vi "ALP3 P.vi"(0 "Header Comments":string="This is a C(T) experiment being done in Physics 350.\r\nIt records the decay response of an RC circuit where the capacitance is a strong function of temperature.", 5 "Temperature Control Parameters":T2={"Start Temp"=30.0, "Temp Step"=10.0, "End Temp"=80.0} {"End Temp" format="%.2f"; "Temp Step" format="%.2f"; "Start Temp" format="%.2f"}, 9 "Timing Control Parameters":T1={"N cycles for averaging"=10, "N points per measurment"=1000, "Measurment time interval"=2e-05} {"Measurment time interval" format="%.2e"}, 11 "error in":errorcluster) -> (3 "Proceed":bool, 4 "data file path out":path, 6 "Temp Array":dbl[](array[numeric]), 10 "Timing Control Parameters out":T1={"N cycles for averaging"=10, "N points per measurment"=1000, "Measurment time interval"=2e-05} {"Measurment time interval" format="%.2e"}, 14 "Auto Launch Data Viewer at End":bool=TRUE, 15 "error out":errorcluster)   [LabVIEW 2016]
doc: "This vi runs when opened, aslo it can open a file, serach for specific numbers on the file to display them in the interface. Also, creates an array with the initail and final temp, and the temp step specified by the user. It can create a file with the data, it found in the file, includes the time, and it can include extra things that the user may want to include in the file. Also has the auto viewer and the data updates dynamically.\n\nAlexis Lopez\nP350\nCSUSB Physics"
uses:
  typedefs/temp control params.ctl
  typedefs/time control params.ctl
panel:
  in  "reload parameters":bool
  in  "exit":bool
  in  "create file and proceed":bool
  out "File Header":string="This is a C(T) experiment being done in Physics 350.\r\nIt records the decay response of an RC circuit where the capacitance is a strong function of temperature.\n\n2/14/2007\n1:53 PM\r\n\r\nStart temp = 30.0\r\nTemp step = 10.0\r\nEnd temp = 80.0\r\nNum temps = 6\r\nNum avg cycles = 10\r\nNum points per meas = 1000\r\nMeas time interval = 2.00E-5\n\nDDD\n\n"
  out "N temps":i32=6
  in  "Auto Launch Data Viewer at End":bool=TRUE
  # "Alexis Lopez\nP350\nCSUSB Physics"
  # "P350 C(T) Experimental Initialization"
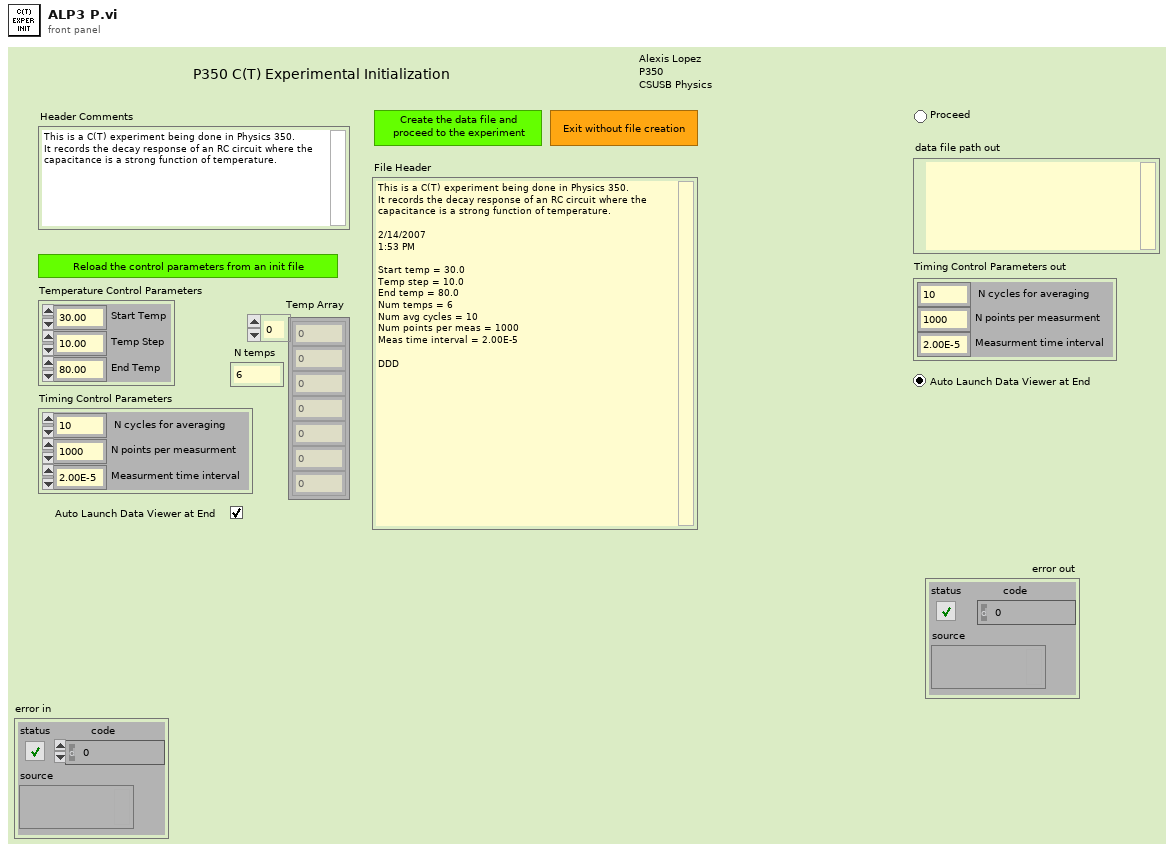
[diagram p1: front panel]
types:
  T1 = typedef "time control params.ctl" = cluster{"N cycles for averaging":i32, "N points per measurment":i32, "Measurment time interval":dbl}
  T2 = typedef "temp control params.ctl" = cluster{"Start Temp":dbl, "Temp Step":dbl, "End Temp":dbl}
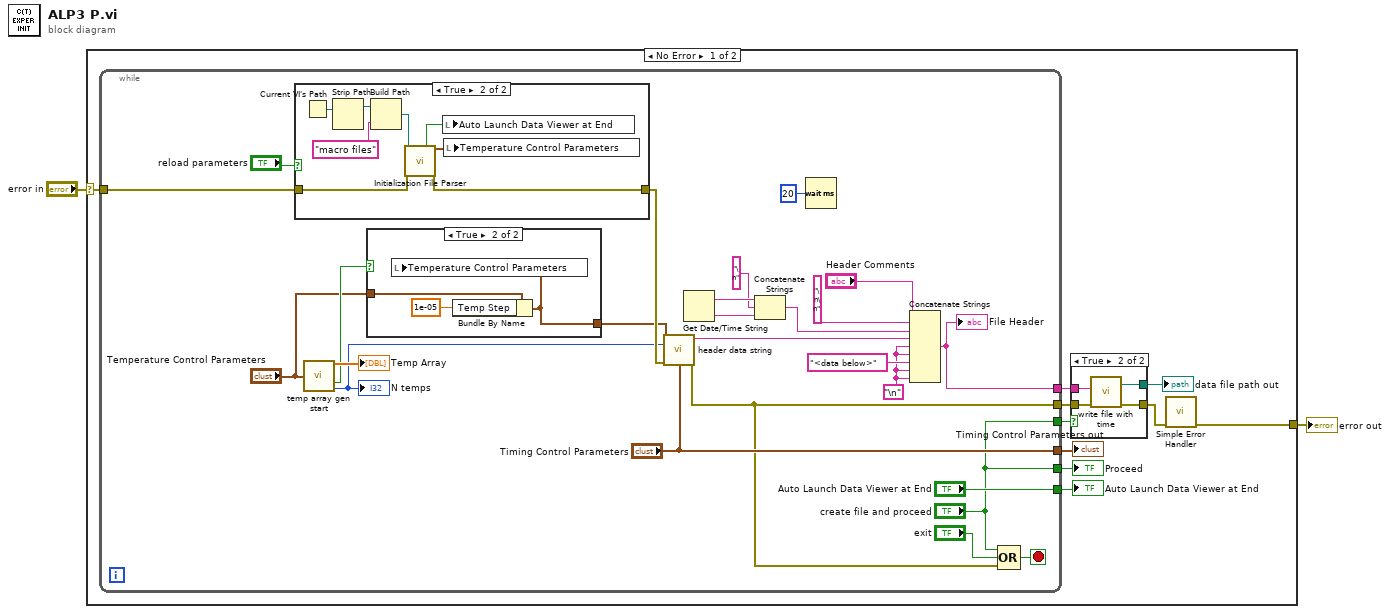
[diagram p0: block diagram]
diagram:
  n1 = case shown="No Error" "error in" {
    selector: "error in" -> [w12 w56]
    tunnel: [w3 w56] -> w1
    frame No Error {
      n2 = while {
        tunnel: [w42] -> w7
        tunnel: ["Auto Launch Data Viewer at End"] -> w10
        tunnel: ["Timing Control Parameters"] -> w11
        tunnel: ["create file and proceed"] -> w4
        tunnel: w12 -> [w34]
        tunnel: ["create file and proceed"] -> w9
        tunnel: [w29] -> w8
        stop <- w31 stop-if-true
        w37 = "\n"
        n3 = case shown="True" "reload parameters" {
          tunnel: w34 -> [w47 w55]
          tunnel: [w47 w54] -> w30
          frame False {
          }
          frame True {
            n4 = Current VI's Path() -> (path=w50:path)
            n5 = Strip Path(path=w50) -> (stripped path=w51:path)  [unwired: 1 out]
            n6 = Build Path(base path=w51, name or relative path="macro files") -> (appended path=w48:path)
            n7 = call "Initialization File Parser.vi"("path in"=w48, "error in"=w55) -> ("Auto Launch Data Viewer at End"=w52:bool, "temp control parameters"=w53:T2, "error out"=w54:errorcluster)  [unwired: 9 in, 2 out]
            n8 = local write "Auto Launch Data Viewer at End"(w52) -> ()
            n9 = local write "Temperature Control Parameters"(w53) -> ()
          }
        }
        n10 = call "temp array gen start.vi"("Temperature Control Parameters"="Temperature Control Parameters") -> ("Temp Array"=→"Temp Array":dbl[], "Warning time step too small"=w27:bool, "N temps"=w28:i32)  [unwired: 12 in]
        "N temps" <- w28
        n11 = case shown="True" w27 {
          tunnel: "Temperature Control Parameters" -> [w43 w46]
          tunnel: [w43 w44] -> w25
          frame False {
          }
          frame True {
            n12 = Bundle By Name(cluster=w46, "Temp Step"=1e-05) -> (w44:T2)
            n13 = local write "Temperature Control Parameters"(w44) -> ()
          }
        }
        n14 = call "header data string.vi"("Temperature Control Parameters"=w25, "N temps"=w28, "error in (no error)"=w30, "Timing Control Parameters"="Timing Control Parameters") -> ("Header string component"=w38:string, "error out"=w29:errorcluster)  [unwired: 10 in]
        n15 = Get Date/Time String() -> (date string=w23:string, time string=w19:string)  [unwired: 3 in]
        n16 = Concatenate Strings(w23, "\n", w19) -> (w20:string)
        n17 = Wait (ms)(milliseconds to wait=u32 20) -> ()  [unwired: 1 out]
        n18 = Concatenate Strings("Header Comments", "\n\n", w20, w38, w37, w37, "<data below>", w37, w37) -> (w42:string)
        "File Header" <- w42
        n19 = Compound Arithmetic op=OR("create file and proceed", "exit", w29) -> (w31:bool)
      }
      "Timing Control Parameters out" <- w11
      "Auto Launch Data Viewer at End" <- w10
      "Proceed" <- w9
      n20 = case shown="True" w4 {
        tunnel: [w13 w17] -> w5
        tunnel: w8 -> [w13 w16]
        tunnel: w7 -> [_ w15]
        tunnel: [_ w14] -> w6
        frame False {
        }
        frame True {
          n21 = call "write file with time.vi"("error in"=w16, "data"=w15) -> ("error out"=w17:errorcluster, "data file path out"=w14:path)  [unwired: 8 in]
        }
      }
      "data file path out" <- w6
      n22 = call <vilib>:"Simple Error Handler.vi"("error in (no error)"=w5) -> ("error out"=w3:errorcluster)  [unwired: 4 in, 4 out]
    }
    frame Error {
    }
  }
  "error out" <- w1
